vi "UI SaveAs Config.vi"(8 "error in (no error)":errorcluster, 11 "MainUI in":refnum<class "UI_Top_Customer.lvclass">) -> (0 "error out":errorcluster, 3 "MainUI out":refnum<class "UI_Top_Customer.lvclass">)   [LabVIEW 2021, in "UI_Top_Customer.lvclass"]
uses:
  UI_Top_Customer.lvclass
  C:/Program Files (x86)/National Instruments/LabVIEW 2021/user.lib/John_Lib/AbstractActorTemplate/AbstractActorTemplate/UIActorTop.lvclass
  <vilib>/Utility/miscctls.llb/LVPositionTypeDef.ctl
  UI_Top_Customer.lvclass/UI_Top_Customer.ctl
  5272a4d7-9cc4-427f-9771-8c62a58d321e.vi
  f5f387c3-e03f-4a00-ba87-cc5ddb2ea158.vi
  <vilib>/JDP Science/JSONtext/Next JSON Value.vi
  <vilib>/JDP Science/JSONtext/String Subset.vi
  <vilib>/JDP Science/JSONtext/Parsing/Advance past next JSON Value (inlined COPY).vi
  <vilib>/JDP Science/JSONtext/Parsing/Advance past whitespace.vi
  <vilib>/JDP Science/JSONtext/Parsing/Advance past String.vi
  <vilib>/JDP Science/JSONtext/Parsing/Advance past Number.vi
  <vilib>/JDP Science/JSONtext/Parsing/Advance past Line Ending.vi
  <vilib>/JDP Science/JSONtext/Variant to JSON Text.vi
  <vilib>/JDP Science/JSONtext/Set Multiple Object Items.vi
  <vilib>/JDP Science/JSONtext/Parsing/Parse Full Path or Item Name.vi
  <vilib>/JDP Science/JSONtext/Parsing/Advance past Array.vi
  <vilib>/JDP Science/JSONtext/Parsing/Advance past Object.vi
  <vilib>/JDP Science/JSONtext/support/Error Cluster From Code.vi
  <vilib>/JDP Science/JSONtext/Offset/Find Item Locations by Path.vi
  <vilib>/JDP Science/JSONtext/JSON text to Variant.vi
  <vilib>/JDP Science/JSONtext/LVClass Serializer/JSONtext LVClass Serializer.lvclass
  <userlib>/John_Lib/AbstractActorTemplate/AbstractActorTemplate/UIActorTop.lvclass
  <userlib>/FTools/JSON Pretty Printer/JSON Pretty Printer.lvlib
  <vilib>/JDP Science/JSONtext/JSONtext.lvlib
  C:/Program Files (x86)/National Instruments/LabVIEW 2021/vi.lib/ActorFramework/Actor/Actor.lvclass
  Z:/Test_Data_Management - Copy/LV Sources/UI_Top_Customer/UI_Top_Customer.lvclass
  C:/Program Files (x86)/National Instruments/LabVIEW 2021/user.lib/John_Lib/Interfaces/InsertMainSubPanel/InsertMainSubPanel.lvclass
panel:
  out "<JSON> 2":string caption="<JSON>Item"
  out "Data out 3":T1
  out "<JSON>":string
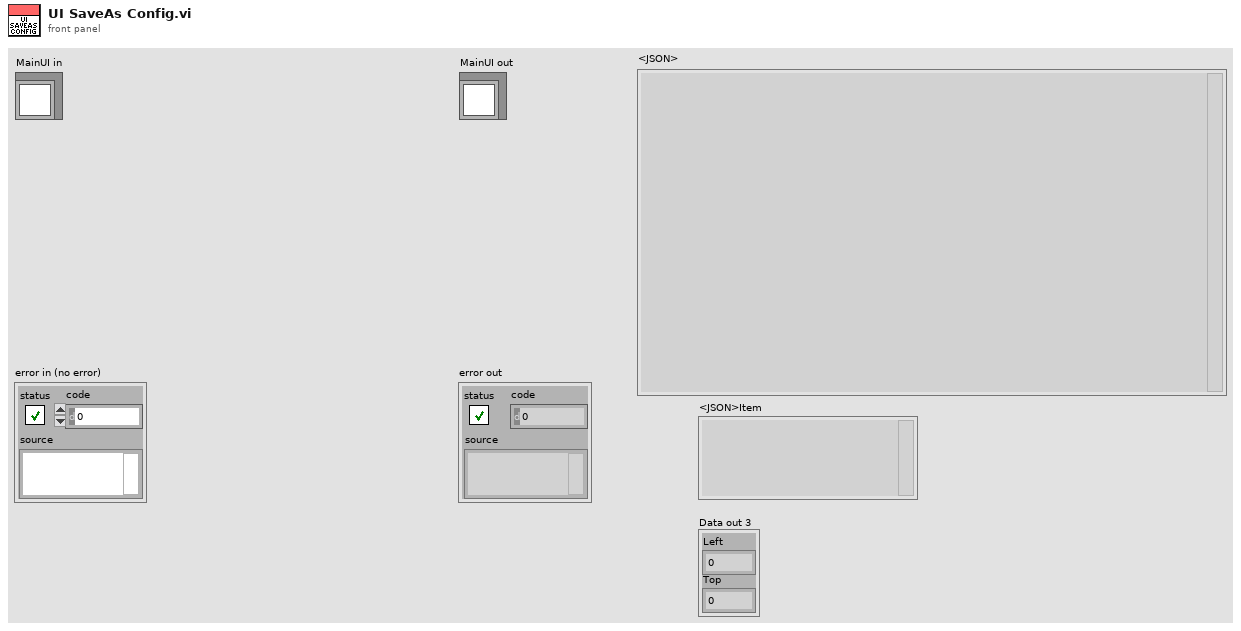
[diagram p1: front panel]
types:
  T1 = typedef "LVPositionTypeDef.ctl" = cluster{"Left":i32, "Top":i32}
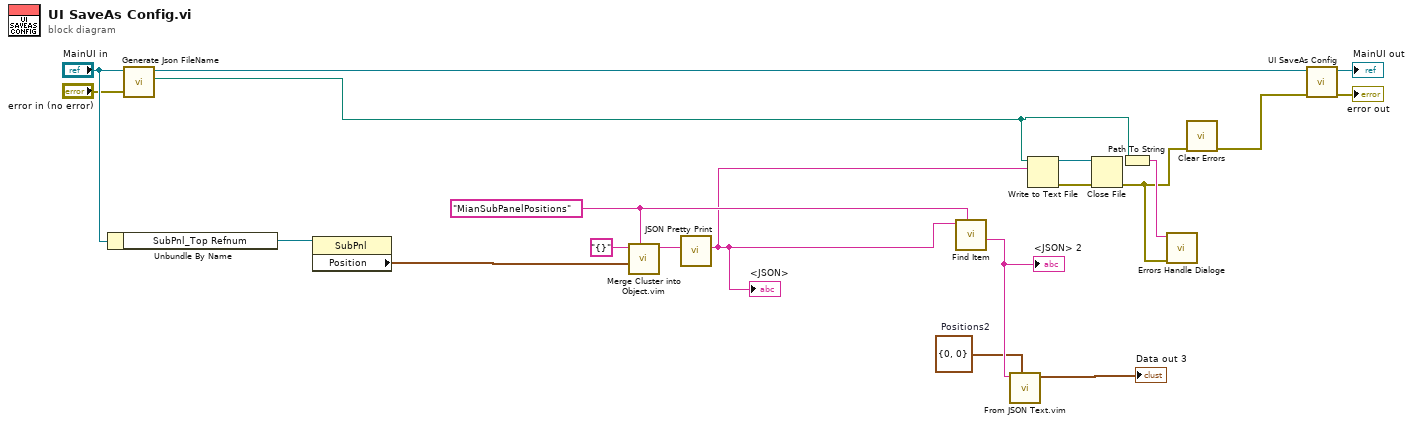
[diagram p0: block diagram]
diagram:
  w15 = T1 {"Left"=0, "Top"=0}  # Positions2
  w11 = "MianSubPanelPositions" ("$Path or Item Name")
  n1 = Unbundle By Name("MainUI in") -> ("SubPnl_Top Refnum"=w18:refnum<vi>)
  n2 = call <userlib>:"Generate Json FileName.vi"("error in (no error)"="error in (no error)", "UIActorTop in"="MainUI in") -> ("Json File path"=w3:path, "UIActorTop out"=w4:refnum<class "UI_Top_Customer.lvclass">)  [unwired: 7 in, 1 out]
  n3 = property class="SubPnl"(reference=w18) -> ("Position"=w13:T1)  [unwired: 1 in, 2 out]
  n4 = call "Merge Cluster into Object.vim"("$Path or Item Name"=w11, "Any Cluster"=w13, "JSON"="{}") -> ("<JSON>"=w12:string)  [unwired: 6 in, 1 out]
  n5 = call <userlib>:"JSON Pretty Print.vi"("JSON String"=w12) -> ("JSON Pretty Print Format"=w10:string)  [unwired: 9 in, 1 out]
  "<JSON>" <- w10
  n6 = call <vilib>:"Find Item.vi"("$Path or Item Name"=w11, "JSON"=w10) -> ("<JSON>"=w16:string)  [unwired: 6 in, 3 out]
  "<JSON> 2" <- w16
  n7 = call "From JSON Text.vim"("Data Type and Default Value"=w15, "JSON"=w16) -> ("Data out"=→"Data out 3":T1)  [unwired: 8 in, 1 out]
  n8 = Write to Text File(file (use dialog)=w3, text=w10) -> (refnum out=w9:refnum<file>, error out=w8:errorcluster)  [unwired: 2 in, 1 out]
  n9 = Close File(refnum=w9, error in=w8) -> (error out=w1:errorcluster)  [unwired: 1 out]
  n10 = Path To String(path=w3) -> (string=w2:string)
  n11 = call <userlib>:"Errors Handle Dialoge.vi"("error in (no error)"=w1, "Message"=w2) -> ()  [unwired: 8 in, 2 out]
  n12 = call <vilib>:"Clear Errors.vi"("error in (no error)"=w1) -> ("error out"=w7:errorcluster)  [unwired: 5 in, 1 out]
  n13 = call-parent "UI SaveAs Config.vi"("error in (no error)"=w7, "UIActorTop in"=w4) -> ("error out"=→"error out":errorcluster, "UIActorTop out"=→"MainUI out":refnum<class "UI_Top_Customer.lvclass">)  [unwired: 8 in]
